vi "Valid Teller Metadata.vi"(10 "Teller Metadata":refnum<class "Teller Metadata.lvclass">) -> (2 "Valid Teller Metadata":bool)   [LabVIEW 2020, in "jettl.lvlib"]
uses:
  jettl.lvlib
  Teller Metadata/Teller Metadata.lvclass
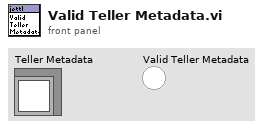
[diagram p1: front panel]
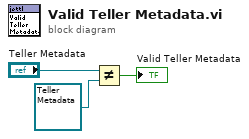
[diagram p0: block diagram]
diagram:
  n1 = Not Equal?(x="Teller Metadata", y=refnum<class "Teller Metadata.lvclass"> refnum) -> (x != y?=→"Valid Teller Metadata":bool)
